vi "readTimeDriven.vi"(8 "Error In":errorcluster, 10 "#cicles":i32, 11 "FGV_data":T2) -> (0 "Error Out":errorcluster, 1 "EOF":bool, 2 "data":T1[](array[typedef]), 3 "FGV_data out":T2)   [LabVIEW 2018]
uses:
  FGV_data.ctl
  Config/config_data.ctl
  AE/timeDriven_data.ctl
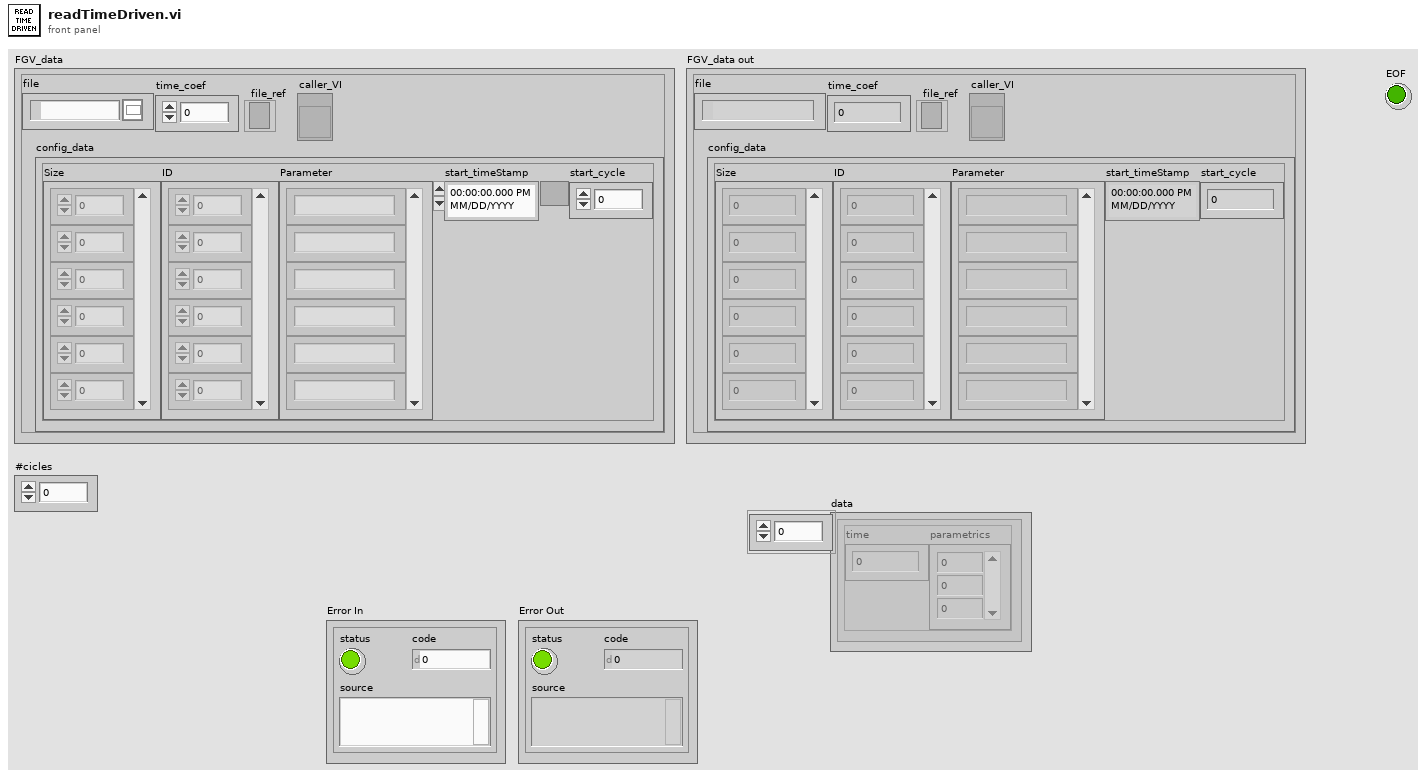
[diagram p1: front panel]
types:
  T1 = typedef "timeDriven_data.ctl" = cluster{"time":dbl, "parametrics":i16[]}
  T2 = typedef "FGV_data.ctl" = cluster{"file":path, "time_coef":dbl, "config_data":T3, "file_ref":refnum<file>, "caller_VI":refnum<vi>}
  T3 = typedef "config_data.ctl" = cluster{"Size":i32[], "ID":u8[], "Parameter":string[], "start_timeStamp":timestamp, "start_cycle":u64}
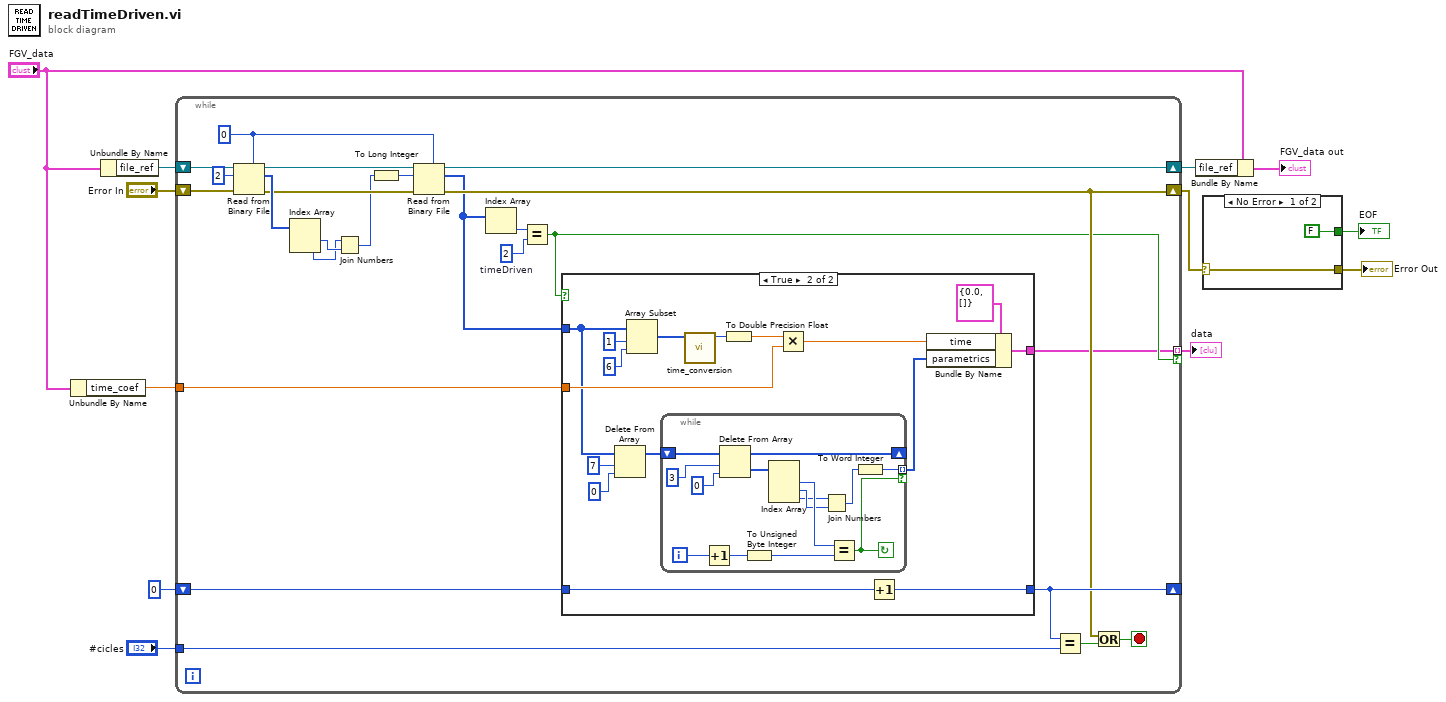
[diagram p0: block diagram]
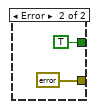
[diagram p3: hidden frame]
diagram:
  n1 = Unbundle By Name("FGV_data") -> ("time_coef"=w7:dbl)
  n2 = Unbundle By Name("FGV_data") -> ("file_ref"=w12:refnum<file>)
  n3 = while {
    shift-right: [w16] -> w4
    shift-left: "Error In" -> [w28]
    tunnel: [w13] -> w1 mode=indexing if=w14
    shift-right: [w23] -> w10
    shift-left: w12 -> [w36]
    tunnel: w7 -> [w22]
    shift-right: [w20] -> _
    shift-left: 0 ("index") -> [w21]
    tunnel: "#cicles" -> [w19]
    stop <- w17 stop-if-true
    w25 = u8 2  # timeDriven
    w31 = u8 0
    n4 = Read from Binary File(5:w31, 8:w28, 10:2 ("count (1)"), 11:w36) -> (0:w32:errorcluster, 2:w34:u8[], 3:w33:refnum<file>)  [unwired: 2 in, 1 out]
    n5 = Index Array(array=w34) -> (element #1=w30:u8, element #2=w29:u8)  [unwired: 2 in]
    n6 = Join Numbers(hi=w29, lo=w30) -> ((hi.lo)=w27:u16)
    n7 = To Long Integer(number=w27) -> (32bit integer=w26:i32)
    n8 = Read from Binary File(5:w31, 8:w32, 10:w26, 11:w33) -> (0:w16:errorcluster, 2:w15:u8[], 3:w23:refnum<file>)  [unwired: 2 in, 1 out]
    n9 = Index Array(array=w15) -> (element=w24:u8)  [unwired: 1 in]
    n10 = Equal?(x=w24, y=w25) -> (x = y?=w14:bool)
    n11 = case shown="True" w14 {
      tunnel: w15 -> [_ w42]
      tunnel: w22 -> [_ w43]
      tunnel: [w37 w48] -> w20
      tunnel: w21 -> [w37 w47]
      tunnel: [_ w38] -> w13
      frame False {
      }
      frame True {
        n12 = Delete From Array(array=w42, length=7 ("inicial"), index=0) -> (array with subset deleted=w49:u8[])  [unwired: 1 out]
        n13 = Array Subset(array=w42, index=1, length=6) -> (w45:u8[])
        n14 = while {
          shift-right: [w67] -> _
          shift-left: w49 -> [w65]
          tunnel: [w54] -> w39 mode=indexing if=w58
          i -> [w63]
          stop <- w58 continue-if-true
          n15 = Increment(x=w63) -> (x+1=w61:i32)
          n16 = Delete From Array(array=w65, length=3, index=0) -> (deleted portion=w59:u8[], array with subset deleted=w67:u8[])
          n17 = To Unsigned Byte Integer(number=w61) -> (unsigned 8bit integer=w60:u8)
          n18 = Index Array(array=w59) -> (element #1=w62:u8, element #2=w57:u8, element #3=w56:u8)  [unwired: 3 in]
          n19 = Join Numbers(hi=w56, lo=w57) -> ((hi.lo)=w55:u16)
          n20 = Equal?(x=w62, y=w60) -> (x = y?=w58:bool)
          n21 = To Word Integer(number=w55) -> (16bit integer=w54:i16)
        }
        n22 = call "time_conversion.vi"("array_time"=w45) -> ("time_U64"=w44:u64)  [unwired: 10 in]
        n23 = To Double Precision Float(number=w44) -> (double precision float=w46:dbl)
        n24 = Multiply(x=w46, y=w43) -> (x*y=w40:dbl)
        n25 = Increment(x=w47) -> (x+1=w48:i32)
        n26 = Bundle By Name(cluster=T1 {"time"=0.0, "parametrics"=[]} ("timeDriven_data"), "time"=w40, "parametrics"=w39) -> (w38:T1)
      }
    }
    n27 = Equal?(x=w20, y=w19) -> (x = y?=w18:bool)
    n28 = Or(x=w16, y=w18) -> (x .or. y?=w17:bool)
  }
  "data" <- w1
  n29 = Bundle By Name(cluster="FGV_data", "file_ref"=w10) -> (→"FGV_data out":T2)
  n30 = case shown="No Error" w4 {
    selector: w4 -> [w69 _]
    tunnel: [w69 errorcluster {"status"=FALSE, "code"=0, "source"=""} ("error IO")] -> w3
    tunnel: [FALSE ("EOF") TRUE ("EOF")] -> w2
    frame No Error {
    }
    frame Error {
    }
  }
  "Error Out" <- w3
  "EOF" <- w2
